vi "rad_to_deg.vi"(1 "Radians":dbl) -> (0 "Degrees":dbl)   [LabVIEW 2010]
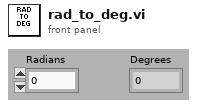
[diagram p1: front panel]
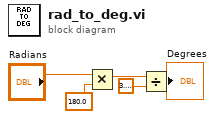
[diagram p0: block diagram]
diagram:
  n1 = Multiply(x="Radians", y=180.0) -> (x*y=w1:dbl)
  n2 = Divide(x=w1, y=3.141592653589793) -> (x/y=→"Degrees":dbl)
